vi "H5Oget_info.vi"(6 "error in (no error)":errorcluster, 9 "HDF5 Ref":T5) -> (0 "error out":errorcluster, 2 "Object Info":T1 {"H5O_hdr_info_t"."mesg"."shared" format="%.0x"; "H5O_hdr_info_t"."mesg"."present" format="%.0x"; "H5O_hdr_info_t"."flags" format="%.0x"; "type" items=["H5O_TYPE_UNKNOWN"=-1, "H5O_TYPE_GROUP"=0, "H5O_TYPE_DATASET"=1, "H5O_TYPE_NAMED_DATATYPE"=2]}, 3 "HDF5 Ref out":T5)   [LabVIEW 2017]
doc: "Retrieves the metadata for an object specified by an identifier."
uses:
  <vilib>/UPVI/lvhdf5/library.llb/HDF5 Ref.ctl
  <vilib>/UPVI/lvhdf5/object.llb/LVH5O_info_t.ctl
  <vilib>/UPVI/lvhdf5/object.llb/H5O_type_t.ctl
  <vilib>/UPVI/lvhdf5/object.llb/H5O_hdr_info_t.ctl
  <vilib>/UPVI/lvhdf5/library.llb/H5_ih_info_t.ctl
  <vilib>/UPVI/lvhdf5/object.llb/H5O_info_t.ctl
  <vilib>/UPVI/lvhdf5/hdf5.dll
panel:
  # "LVHDF5 Toolkit\nCopyright (c) 2005-2013 by Jason D. Sommerville\nCopyright (c) 2014-2015 by UPVI, LLC.\n\nThis use and distribution of this file is governed by the terms found in \nLICENSE.txt distributed with this toolkit and installed at\n <user.lib>\\_lvhdf5\\LICENSE.txt"
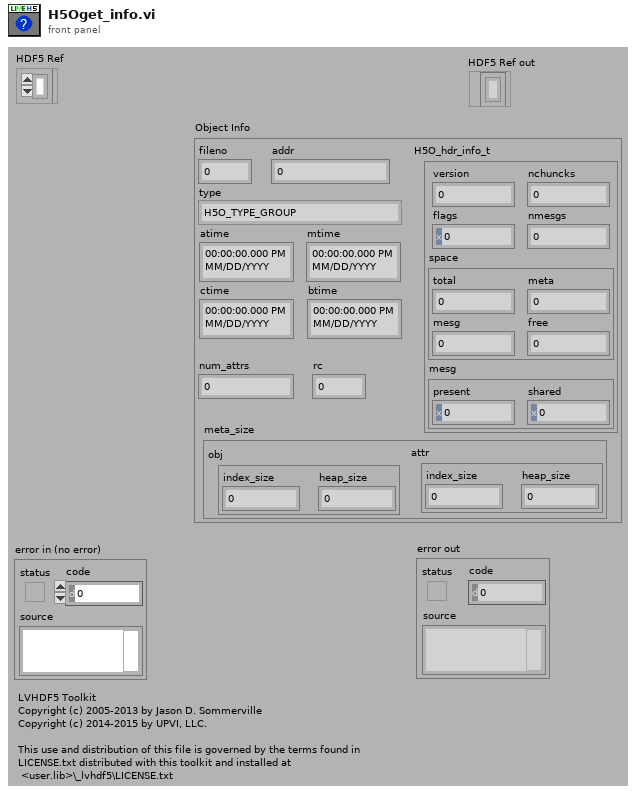
[diagram p1: front panel]
types:
  T1 = typedef "LVH5O_info_t.ctl" = cluster{"fileno":u32, "addr":u64, "type":T2, "rc":u32, "atime":timestamp, "mtime":timestamp, "ctime":timestamp, "btime":timestamp, "num_attrs":i64, "H5O_hdr_info_t":T3, "meta_size":cluster{"obj":T4, "attr":T4}}
  T2 = typedef "H5O_type_t.ctl" = i32
  T3 = typedef "H5O_hdr_info_t.ctl" = cluster{"version":u32, "nmesgs":u32, "nchuncks":u32, "flags":u32, "space":cluster{"total":u64, "meta":u64, "mesg":u64, "free":u64}, "mesg":cluster{"present":u64, "shared":u64}}
  T4 = typedef "H5_ih_info_t.ctl" = cluster{"index_size":u64, "heap_size":u64}
  T5 = typedef "HDF5 Ref.ctl" = refnum<k1>
  T6 = typedef "H5O_info_t.ctl" = cluster{"fileno":u32, "unused":u32, "addr":u64, "type":T2, "rc":u32, "atime":i64, "mtime":i64, "ctime":i64, "btime":i64, "num_attrs":i64, "H5O_hdr_info_t":T3, "meta_size":cluster{"obj":T4, "attr":T4}}
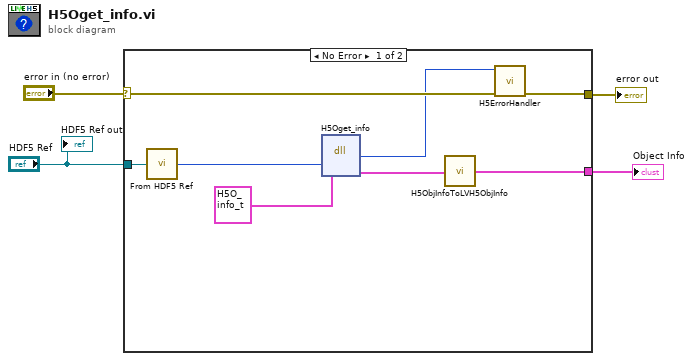
[diagram p0: block diagram]
diagram:
  n1 = case shown="No Error" "error in (no error)" {
    selector: "error in (no error)" -> [w12 w13]
    tunnel: [w11 w13] -> w3
    tunnel: "HDF5 Ref" -> [w10 _]
    tunnel: [w5 _] -> w1
    frame No Error {
      n2 = call <vilib>:"From HDF5 Ref.vi"("HDF5 Ref"=w10) -> ("I32"=w9:i32)
      n3 = dll-call lib="C:/Program Files/National Instruments/LabVIEW 2017/vi.lib/UPVI/lvhdf5/hdf5.dll" fn="H5Oget_info"("loc_id"=w9, "info"=T6 {"fileno"=0, "unused"=0, "addr"=0, "type"=0, "rc"=0, "atime"=0, "mtime"=0, "ctime"=0, "btime"=0, "num_attrs"=0, "H5O_hdr_info_t"={"version"=0, "nmesgs"=0, "nchuncks"=0, "flags"=0, "space"={"total"=0, "meta"=0, "mesg"=0, "free"=0}, "mesg"={"present"=0, "shared"=0}}, "meta_size"={"obj"={"index_size"=0, "heap_size"=0}, "attr"={"index_size"=0, "heap_size"=0}}}) -> ("return type"=w8:i32, "info"=w6:T6)  [unwired: 4 in, 2 out]
      n4 = call <vilib>:"H5ObjInfoToLVH5ObjInfo.vi"("H5O_info_t"=w6) -> ("LVH5O_info_t"=w5:T1)
      n5 = call <vilib>:"H5ErrorHandler.vi"("error in (no error)"=w12, "herr_t"=w8) -> ("error out"=w11:errorcluster)  [unwired: 3 in, 4 out]
    }
    frame Error {
    }
  }
  "error out" <- w3
  "Object Info" <- w1
  "HDF5 Ref out" <- "HDF5 Ref"
